vi "test_multiple_connections.vi"(8 "error in (no error)":errorcluster caption="エラー入力（エラーなし）", 11 "Hardware":T1={"SQUID"={"port"="", "Flux constant"={"X"=8.34e-05, "Y"=-8.11e-05, "Z"=-4.28e-05}, "X"=10, "Y"=10, "Z"=10}, "Sample Handler"={"port"="", "BG 1"=-82132.0, "BG 2"=-22571.0, "Sensor"=-74765.0, "AF 1"=-51160.0, "AF 2"=-123198.0, "Home (relative to limit switch)"=989.0}, "Degausser"={"port"="", "Ramp rate"=3.0, "Tracking timeout (sec)"=60.0, "Communication Delays"=350.0, "Maximum field (Oe)"=1200.0}, "ARM Unit"={"port"=""}, "IRM Unit（未実装）"={"port"=""}, "Robot"={"port"=""}} {"SQUID"."Z" items=["1 Hz"=1, "10 Hz"=10, "100 Hz"=100, "WB"=0]; "SQUID"."Y" items=["1 Hz"=1, "10 Hz"=10, "100 Hz"=100, "WB"=0]; "SQUID"."X" items=["1 Hz"=1, "10 Hz"=10, "100 Hz"=100, "WB"=0]}) -> (0 "error out":errorcluster caption="エラー出力")   [LabVIEW 2017]
uses:
  <vilib>/Instr/_visa.llb/VISA Configure Serial Port (Instr).vi
  controls/XYZ_Data.ctl
  controls/SQUID_filter.ctl
  controls/SQUID_configuration.ctl
  controls/SampleHandler_configuration.ctl
  controls/Degausser_configuration.ctl
  controls/HW Configuration.ctl
panel:
  # "Count"
  # "Relative to Home, Negative=CW"
  # "Filter (未実装）"
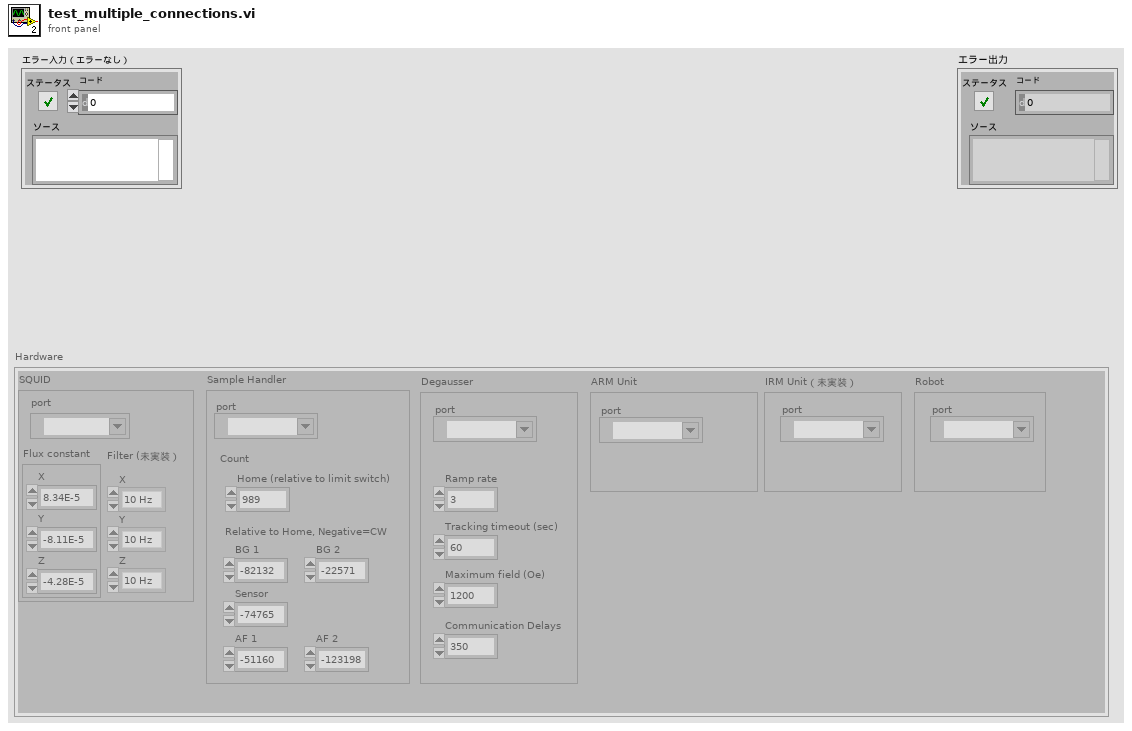
[diagram p1: front panel]
types:
  T1 = typedef "HW Configuration.ctl" = cluster{"SQUID":T2, "Sample Handler":T5, "Degausser":T6, "ARM Unit":cluster{"port":refnum<visa-resource-name>}, "IRM Unit（未実装）":cluster{"port":refnum<visa-resource-name>}, "Robot":cluster{"port":refnum<visa-resource-name>}}
  T2 = typedef "SQUID_configuration.ctl" = cluster{"port":refnum<visa-resource-name>, "Flux constant":T3, "X":T4, "Y":T4, "Z":T4}
  T3 = typedef "XYZ_Data.ctl" = cluster{"X":dbl, "Y":dbl, "Z":dbl}
  T4 = typedef "SQUID_filter.ctl" = u16
  T5 = typedef "SampleHandler_configuration.ctl" = cluster{"port":refnum<visa-resource-name>, "BG 1":dbl, "BG 2":dbl, "Sensor":dbl, "AF 1":dbl, "AF 2":dbl, "Home (relative to limit switch)":dbl}
  T6 = typedef "Degausser_configuration.ctl" = cluster{"port":refnum<visa-resource-name>, "Ramp rate":dbl, "Tracking timeout (sec)":dbl, "Communication Delays":dbl, "Maximum field (Oe)":dbl}
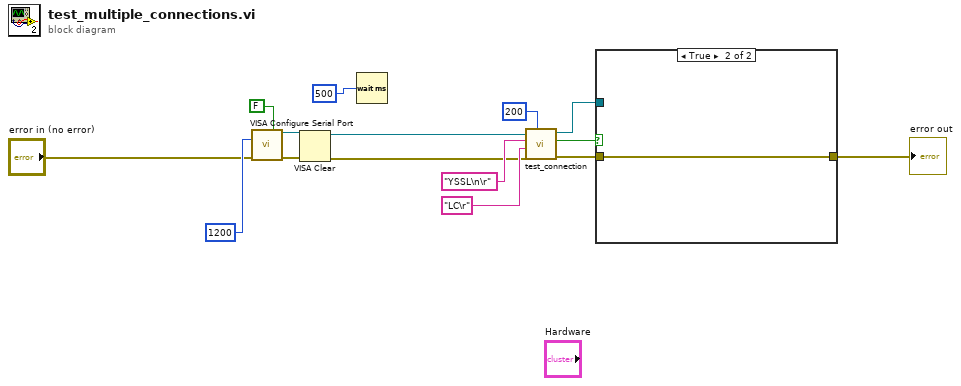
[diagram p0: block diagram]
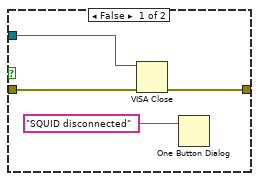
[diagram p2: hidden frame]
diagram:
  n1 = call-poly "VISA Configure Serial Port"("Enable Termination\nChar (T)"=FALSE, "baud rate (9600)"=1200, "error in (no error)"="error in (no error)") -> ("VISA resource name"=w2:refnum<visa-resource-name>, "VISA resource name out"=w9:refnum<visa-resource-name>, "error out"=w8:errorcluster)  [unwired: 10 in]
  n2 = VISA Clear(VISA resource name=w9, error in (no error)=w8) -> (VISA resource name out=w7:refnum<visa-resource-name>, error out=w6:errorcluster)
  n3 = Wait (ms)(milliseconds to wait=500) -> ()  [unwired: 1 out]
  n4 = call "test_connection.vi"("文字送信間隔 (500 ms)"=200, "error in (no error)"=w6, "想定レスポンス"="LC\r", "コマンド"="YSSL\n\r", "VISAリソース名"=w7) -> ("error out"=w12:errorcluster, "一致？"=w1:bool, "VISAリソース名 （出力）"=w11:refnum<visa-resource-name>)  [unwired: 3 in, 1 out]
  n5 = case shown="TRUE" w1 {
    tunnel: w12 -> [w20 w21]
    tunnel: w11 -> [w19 _]
    tunnel: [w17 w21] -> w3
    frame False {
      n6 = VISA Close(VISA resource name=w19, error in (no error)=w20) -> (error out=w17:errorcluster)
      n7 = One Button Dialog(message="SQUID disconnected") -> ()  [unwired: 1 in, 1 out]
    }
    frame True {
    }
  }
  "error out" <- w3
